vi "Table Stage Processor.vi"() -> ()   [LabVIEW 2018]
uses:
  Controls/QueueNames.ctl
  Controls/Queue Manager Actions.ctl
  Controls/MessagePacket.ctl
  Hardware Mfg/Thorlabs Translation Stages/Controls/Motion Translation Module Control.ctl
  Controls/Set Get Controls.ctl
  Controls/FGV Actions.ctl
  Hardware Mfg/Main Scan Processor Status.vi
  Controls/Translation Stage Types.ctl
  Hardware Mfg/Thorlabs Translation Stages/Controls/Translation Stage Cluster.ctl
panel:
  in  "error out":errorcluster
  out "Processor Error Out":errorcluster
  out "Cluster":cluster{"X":T1, "Y":T1, "Z":T1}
  out "Message":string
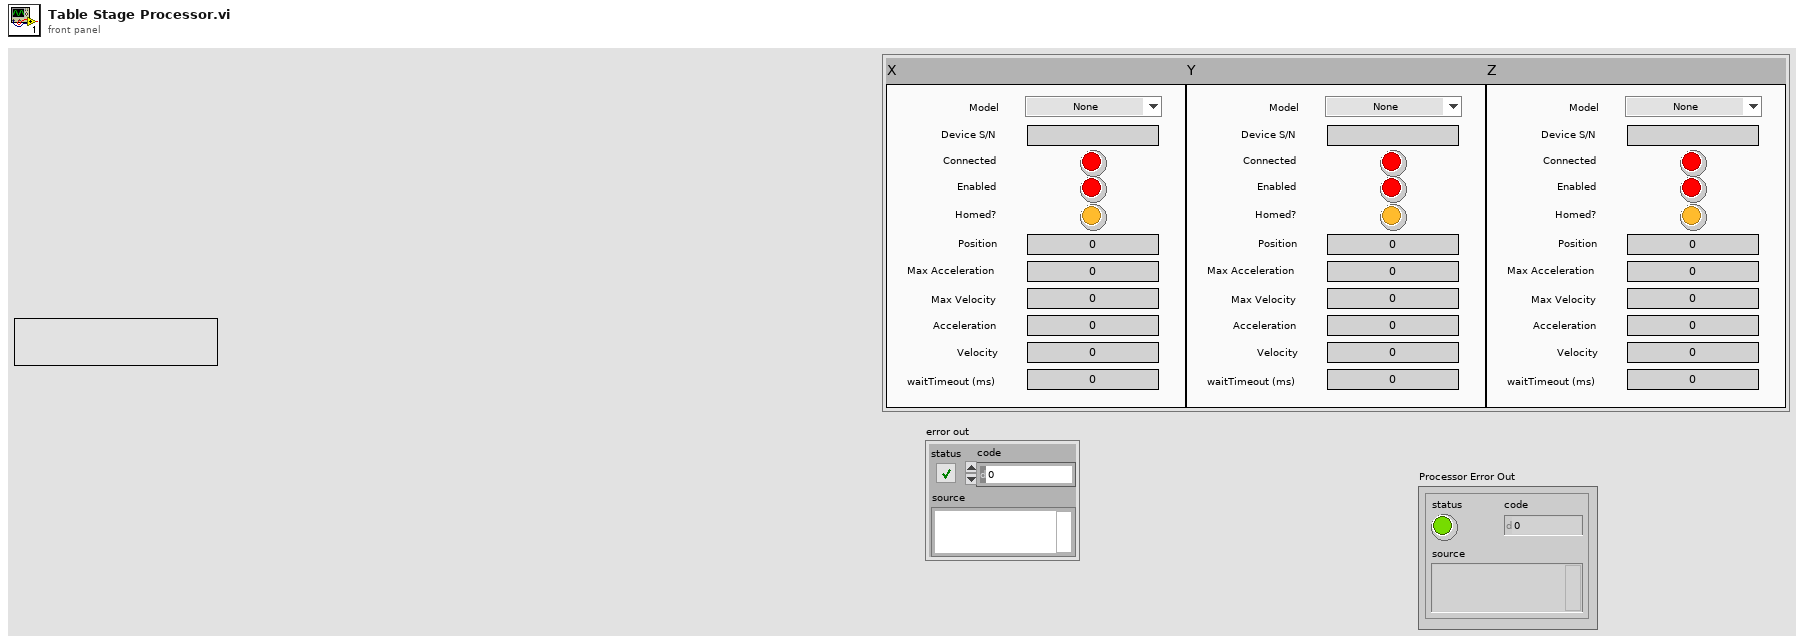
[diagram p1: front panel]
types:
  T1 = typedef "Translation Stage Cluster.ctl" = cluster{"Position":dbl, "Is.Enabled?":bool, "Is.Connected?":bool, "Device SN":string, "AccelerationMaximum":dbl, "VelocityMaximum":dbl, "Acceleration":dbl, "Velocity":dbl, "waitTimeout (ms)":i32, "Model":T2, "Is.Homed?":bool}
  T2 = typedef "Translation Stage Types.ctl" = enum16{"None", "Thorlabs LTS", "Thorlabs MLJ"}
  T3 = typedef "Queue Manager Actions.ctl" = enum16{"Init", "Enqueue", "Enqueue All", "Preview Queue", "Dequeue", "Get Status", "Flush Queue", "Flush All Queues", "Release All Queues", "Release Queue", "Enqueue at Opposite End"}
  T4 = typedef "MessagePacket.ctl" = cluster{"Message":string, "Parameter":variant}
  T5 = typedef "FGV Actions.ctl" = enum16{"Init", "Set", "Get", "Clear"}
  T6 = typedef "Set Get Controls.ctl" = enum16{"Set", "Get"}
  T7 = typedef "Motion Translation Module Control.ctl" = enum16{"Init", "Home", "Status", "Velocity/Accel", "Position", "Jog", "Stop", "Uninit", "Enable", "Disable"}
  T8 = typedef "QueueNames.ctl" = enum16{"Main GUI", "Main Scan Processor", "Main Display", "Main Table Stage GUI", "Main Table Stage Proc.", "Scan Engine", "Vibratome GUI", "Vibratome Processor", "Slice Engine", "Table Stage Processor"}
  T9 = cluster{"X Stage":T1, "Y Stage":T1, "Z Stage":T1}
  T10 = typedef "System Parameters.ctl" = cluster{"Optical /HW Parameters":cluster{"Focal Length [mm]":dbl, "Scan Lens EFL[mm]":dbl, "Tube Lens EFL[mm]":dbl, "Galvo V Range (+/-)":dbl, "Galvo Max Half Angle [Deg]":dbl, "Max Galvo Range[%]":dbl}, "Vibratome":cluster{"Z Bottom [mm]":dbl, "Pre Cut Dwell [s]":dbl, "Blade Frequency [RPM]":u16, "Slice Speed [mm/s]":dbl, "Post Cut Dwell [s]":dbl, "Ramp Time [s]":dbl, "Start X [mm]":dbl, "Start Y [mm]":dbl, "Slice Length [mm]":dbl, "Slice Axis":enum16{"X Axis", "Y Axis", "Z Axis"}, "Controller VISA Ref":refnum<visa-resource-name>}, "Table Stages":cluster{"X Stage":T1, "Y Stage":T1, "Z Stage":T1}, "Imaging Parameter":cluster{"Raster Scan Direction":T11, "Pixel Dwell Time [Clock Cycles]":u16, "Flyback Time [Clock Cycles]":u16, "XY Center [um]":cluster{"X":dbl, "Y":dbl}, "Pixel Step Size [um]":dbl, "XY Image Resolution":enum16{"32 x 32", "64 x 64", "128 x 128", "256 x 256", "512 x 512", "1024 x 1024", "2048 x 2048"}, "Custom":bool, "Custom Size":cluster{"X":u16, "Y":u16}, "Line Averages":u8}}
  T11 = typedef "Scan Direction.ctl" = enum16{"Uni Directional", "Bi Directional", "None"}
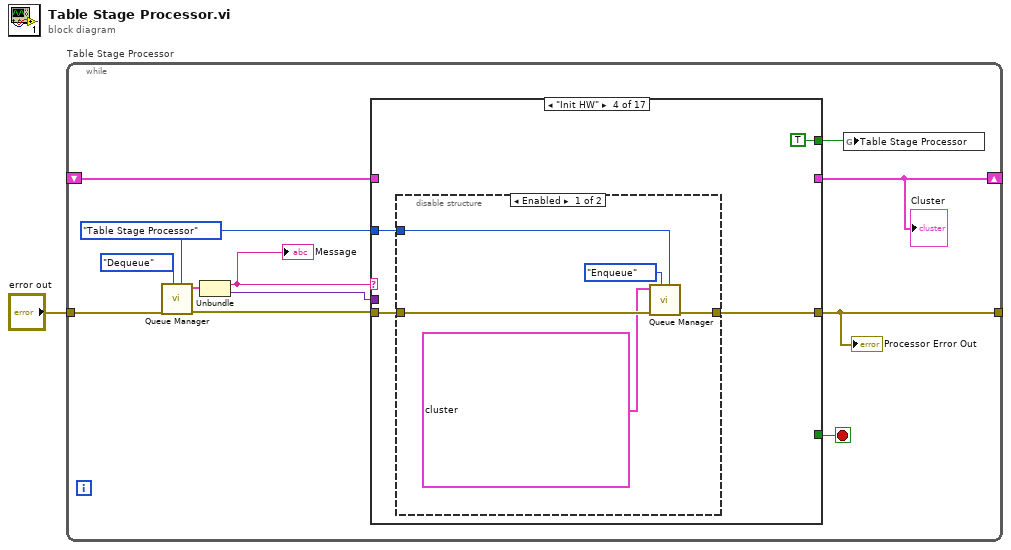
[diagram p0: block diagram]
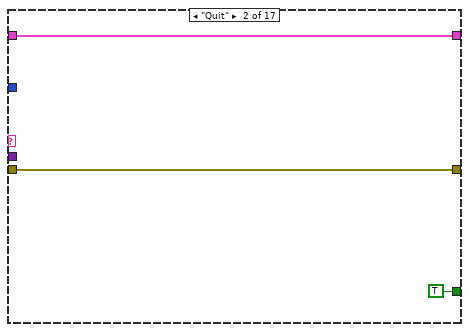
[diagram p3: hidden frame]
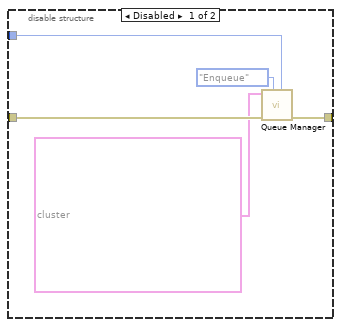
[diagram p5: hidden frame]
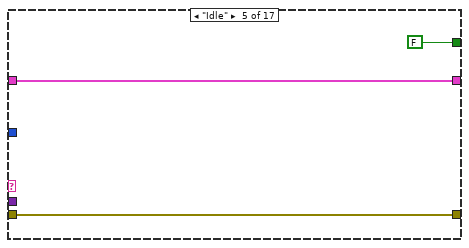
[diagram p7: hidden frame]
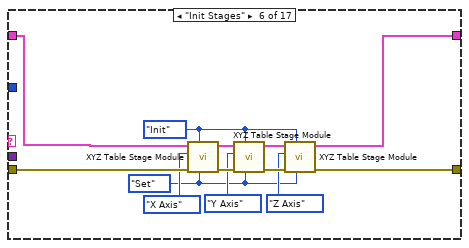
[diagram p8: hidden frame]
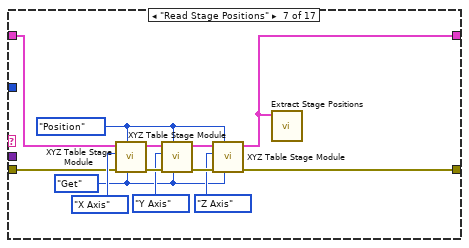
[diagram p9: hidden frame]
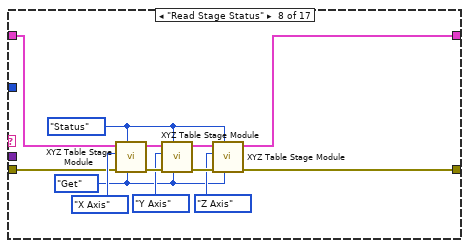
[diagram p10: hidden frame]
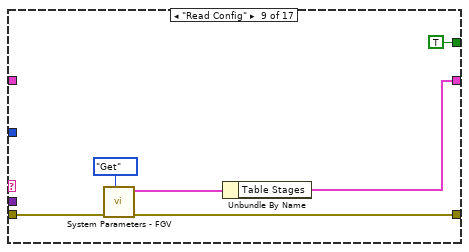
[diagram p11: hidden frame]
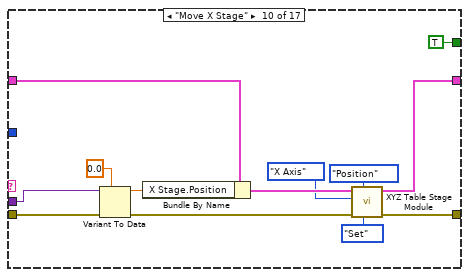
[diagram p12: hidden frame]
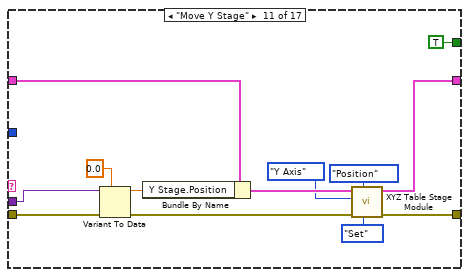
[diagram p13: hidden frame]
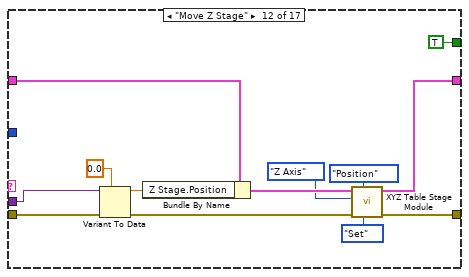
[diagram p14: hidden frame]
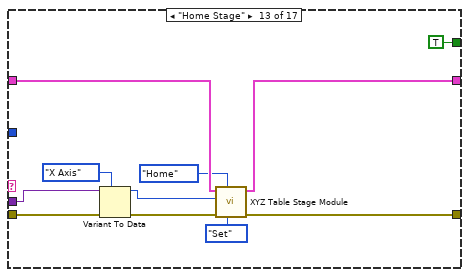
[diagram p15: hidden frame]
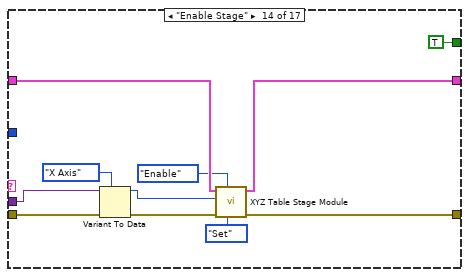
[diagram p16: hidden frame]
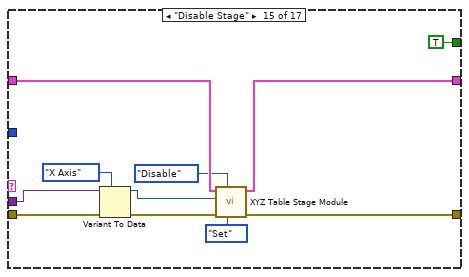
[diagram p17: hidden frame]
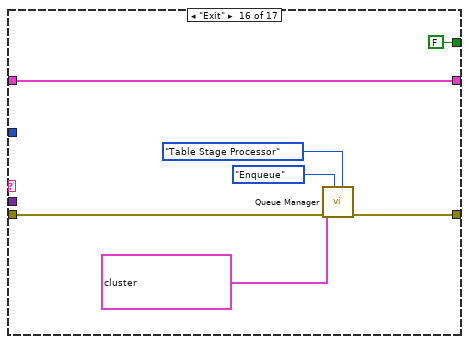
[diagram p18: hidden frame]
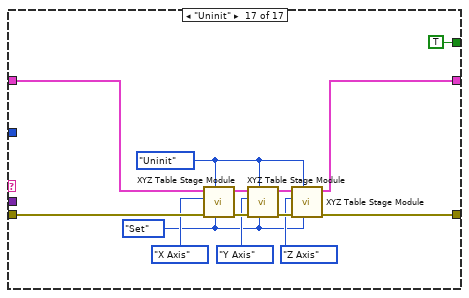
[diagram p19: hidden frame]
diagram:
  n1 = while "Table Stage Processor" {
    tunnel: "error out" -> [w12]
    tunnel: [w13] -> _
    shift-right: [w5] -> _
    shift-left: _ -> [w6]
    stop <- w8 stop-if-true
    w3 = QueueNames."Table Stage Processor" ("Queue Name")
    n2 = call "Queue Manager.vi"("Queue Name"=w3, "Action"=Queue_Manager_Actions."Dequeue", "Error In"=w12) -> ("Error Out"=w4:errorcluster, "Message Packet [Out]"=w11:T4)  [unwired: 4 in, 3 out]
    n3 = Unbundle(w11) -> ("Message"=w10:string, "Parameter"=w9:variant)
    "Message" <- w10
    n4 = case shown="\"Init HW\"" w10 {
      tunnel: w4 -> [w15 w17 w21 w31 w40 w52 w56 w69 w85 w98 w111 w124 w135 w146 w157 w163 w178]
      tunnel: [w15 w17 w20 w30 w40 w53 w64 w77 w83 w97 w110 w123 w134 w145 w156 w162 w166] -> w13
      tunnel: w9 -> [_ _ _ _ _ _ _ _ _ w95 w108 w121 w132 w143 w154 _ _]
      tunnel: [_ TRUE _ _ _ _ _ _ _ _ _ _ _ _ _ _ _] -> w8
      tunnel: [w14 w18 _ _ w39 w50 w54 w67 w84 w94 w107 w120 w128 w139 w150 w164 w172] -> w5
      tunnel: w6 -> [w14 w18 _ _ w39 w51 w55 w68 _ w90 w103 w116 w129 w140 w151 w164 w175]
      tunnel: w3 -> [_ _ w19 w29 _ _ _ _ _ _ _ _ _ _ _ _ _]
      tunnel: [_ _ _ TRUE FALSE _ _ _ TRUE TRUE TRUE TRUE TRUE TRUE TRUE FALSE TRUE] -> w2
      frame "Unknown", Default {
      }
      frame "Quit" {
      }
      frame "Init" {
        n5 = disable-structure shown="Enabled" {
          disable-tunnel: w21 -> [w26 w27]
          disable-tunnel: [w25 w27] -> w20
          disable-tunnel: w19 -> [w22 _]
          frame Disabled {
            n6 = call "Queue Manager.vi"("Queue Name"=w22, "Action"=Queue_Manager_Actions."Enqueue", "Error In"=w26, "Message Packet Array"=T4[] [{"Message"="Read Config", "Parameter"=variant}, {"Message"="Init Stage HW", "Parameter"=variant}, {"Message"="Read Stage Status", "Parameter"=variant}, {"Message"="Read Stage Positions", "Parameter"=variant}]) -> ("Error Out"=w25:errorcluster)  [unwired: 3 in, 4 out]
          }
          frame Enabled {
          }
        }
      }
      frame "Init HW" {
        n7 = disable-structure shown="Enabled" {
          disable-tunnel: w31 -> [w36 w37]
          disable-tunnel: [w35 w37] -> w30
          disable-tunnel: w29 -> [w32 _]
          frame Enabled {
            n8 = call "Queue Manager.vi"("Queue Name"=w32, "Action"=Queue_Manager_Actions."Enqueue", "Error In"=w36, "Message Packet Array"=T4[] [{"Message"="Read Config", "Parameter"=variant}, {"Message"="Init Stages", "Parameter"=variant}, {"Message"="Read Stage Status", "Parameter"=variant}, {"Message"="Read Stage Positions", "Parameter"=variant}, {"Message"="Idle", "Parameter"=variant}]) -> ("Error Out"=w35:errorcluster)  [unwired: 3 in, 4 out]
          }
          frame Disabled {
          }
        }
      }
      frame "Idle" {
      }
      frame "Init Stages" {
        w41 = Set_Get_Controls."Set" ("Set/Get")
        w47 = Motion_Translation_Module_Control."Init" ("Action")
        n9 = call "XYZ Table Stage Module.vi"("Set/Get"=w41, "Action"=w47, "Error In"=w52, "Axis"=enum16{"X Axis", "Y Axis", "Z Axis"}."X Axis", "Table Stages"=w51) -> ("Error Out"=w49:errorcluster, "Table Stages Out"=w46:T9)  [unwired: 5 in]
        n10 = call "XYZ Table Stage Module.vi"("Set/Get"=w41, "Action"=w47, "Error In"=w49, "Axis"=enum16{"X Axis", "Y Axis", "Z Axis"}."Y Axis", "Table Stages"=w46) -> ("Error Out"=w48:errorcluster, "Table Stages Out"=w45:T9)  [unwired: 5 in]
        n11 = call "XYZ Table Stage Module.vi"("Set/Get"=w41, "Action"=w47, "Error In"=w48, "Axis"=enum16{"X Axis", "Y Axis", "Z Axis"}."Z Axis", "Table Stages"=w45) -> ("Error Out"=w53:errorcluster, "Table Stages Out"=w50:T9)  [unwired: 5 in]
      }
      frame "Read Stage Positions" {
        w57 = Set_Get_Controls."Get" ("Set/Get")
        w63 = Motion_Translation_Module_Control."Position" ("Action")
        n12 = call "XYZ Table Stage Module.vi"("Set/Get"=w57, "Action"=w63, "Error In"=w56, "Axis"=enum16{"X Axis", "Y Axis", "Z Axis"}."X Axis", "Table Stages"=w55) -> ("Error Out"=w66:errorcluster, "Table Stages Out"=w62:T9)  [unwired: 5 in]
        n13 = call "XYZ Table Stage Module.vi"("Set/Get"=w57, "Action"=w63, "Error In"=w66, "Axis"=enum16{"X Axis", "Y Axis", "Z Axis"}."Y Axis", "Table Stages"=w62) -> ("Error Out"=w65:errorcluster, "Table Stages Out"=w61:T9)  [unwired: 5 in]
        n14 = call "XYZ Table Stage Module.vi"("Set/Get"=w57, "Action"=w63, "Error In"=w65, "Axis"=enum16{"X Axis", "Y Axis", "Z Axis"}."Z Axis", "Table Stages"=w61) -> ("Error Out"=w64:errorcluster, "Table Stages Out"=w54:T9)  [unwired: 5 in]
        n15 = call "Extract Stage Positions.vi"("Table Stages"=w54) -> ()  [unwired: 8 in, 3 out]
      }
      frame "Read Stage Status" {
        w70 = Set_Get_Controls."Get" ("Set/Get")
        w76 = Motion_Translation_Module_Control."Status" ("Action")
        n16 = call "XYZ Table Stage Module.vi"("Set/Get"=w70, "Action"=w76, "Error In"=w69, "Axis"=enum16{"X Axis", "Y Axis", "Z Axis"}."X Axis", "Table Stages"=w68) -> ("Error Out"=w79:errorcluster, "Table Stages Out"=w75:T9)  [unwired: 5 in]
        n17 = call "XYZ Table Stage Module.vi"("Set/Get"=w70, "Action"=w76, "Error In"=w79, "Axis"=enum16{"X Axis", "Y Axis", "Z Axis"}."Y Axis", "Table Stages"=w75) -> ("Error Out"=w78:errorcluster, "Table Stages Out"=w74:T9)  [unwired: 5 in]
        n18 = call "XYZ Table Stage Module.vi"("Set/Get"=w70, "Action"=w76, "Error In"=w78, "Axis"=enum16{"X Axis", "Y Axis", "Z Axis"}."Z Axis", "Table Stages"=w74) -> ("Error Out"=w77:errorcluster, "Table Stages Out"=w67:T9)  [unwired: 5 in]
      }
      frame "Read Config" {
        n19 = call "System Parameters - FGV.vi"("Actions"=FGV_Actions."Get", "Error In"=w85) -> ("Error Out"=w83:errorcluster, "System Parameters"=w82:T10)  [unwired: 8 in]
        n20 = Unbundle By Name(w82) -> ("Table Stages"=w84:T9)
      }
      frame "Move X Stage" {
        n21 = Variant To Data(error in=w98, type=0.0 ("Value"), Variant=w95) -> (data=w89:dbl, error out=w96:errorcluster)
        n22 = Bundle By Name(cluster=w90, "X Stage.Position"=w89) -> (w88:T9)
        n23 = call "XYZ Table Stage Module.vi"("Set/Get"=Set_Get_Controls."Set", "Action"=Motion_Translation_Module_Control."Position", "Error In"=w96, "Axis"=enum16{"X Axis", "Y Axis", "Z Axis"}."X Axis", "Table Stages"=w88) -> ("Error Out"=w97:errorcluster, "Table Stages Out"=w94:T9)  [unwired: 5 in]
      }
      frame "Move Y Stage" {
        n24 = Variant To Data(error in=w111, type=0.0 ("Value"), Variant=w108) -> (data=w102:dbl, error out=w109:errorcluster)
        n25 = Bundle By Name(cluster=w103, "Y Stage.Position"=w102) -> (w101:T9)
        n26 = call "XYZ Table Stage Module.vi"("Set/Get"=Set_Get_Controls."Set", "Action"=Motion_Translation_Module_Control."Position", "Error In"=w109, "Axis"=enum16{"X Axis", "Y Axis", "Z Axis"}."Y Axis", "Table Stages"=w101) -> ("Error Out"=w110:errorcluster, "Table Stages Out"=w107:T9)  [unwired: 5 in]
      }
      frame "Move Z Stage" {
        n27 = Variant To Data(error in=w124, type=0.0 ("Value"), Variant=w121) -> (data=w115:dbl, error out=w122:errorcluster)
        n28 = Bundle By Name(cluster=w116, "Z Stage.Position"=w115) -> (w114:T9)
        n29 = call "XYZ Table Stage Module.vi"("Set/Get"=Set_Get_Controls."Set", "Action"=Motion_Translation_Module_Control."Position", "Error In"=w122, "Axis"=enum16{"X Axis", "Y Axis", "Z Axis"}."Z Axis", "Table Stages"=w114) -> ("Error Out"=w123:errorcluster, "Table Stages Out"=w120:T9)  [unwired: 5 in]
      }
      frame "Home Stage" {
        n30 = Variant To Data(error in=w135, type=enum16{"X Axis", "Y Axis", "Z Axis"}."X Axis" ("Axis"), Variant=w132) -> (data=w130:enum16{"X Axis", "Y Axis", "Z Axis"}, error out=w133:errorcluster)
        n31 = call "XYZ Table Stage Module.vi"("Set/Get"=Set_Get_Controls."Set", "Action"=Motion_Translation_Module_Control."Home", "Error In"=w133, "Axis"=w130, "Table Stages"=w129) -> ("Error Out"=w134:errorcluster, "Table Stages Out"=w128:T9)  [unwired: 5 in]
      }
      frame "Enable Stage" {
        n32 = Variant To Data(error in=w146, type=enum16{"X Axis", "Y Axis", "Z Axis"}."X Axis" ("Axis"), Variant=w143) -> (data=w141:enum16{"X Axis", "Y Axis", "Z Axis"}, error out=w144:errorcluster)
        n33 = call "XYZ Table Stage Module.vi"("Set/Get"=Set_Get_Controls."Set", "Action"=Motion_Translation_Module_Control."Enable", "Error In"=w144, "Axis"=w141, "Table Stages"=w140) -> ("Error Out"=w145:errorcluster, "Table Stages Out"=w139:T9)  [unwired: 5 in]
      }
      frame "Disable Stage" {
        n34 = Variant To Data(error in=w157, type=enum16{"X Axis", "Y Axis", "Z Axis"}."X Axis" ("Axis"), Variant=w154) -> (data=w152:enum16{"X Axis", "Y Axis", "Z Axis"}, error out=w155:errorcluster)
        n35 = call "XYZ Table Stage Module.vi"("Set/Get"=Set_Get_Controls."Set", "Action"=Motion_Translation_Module_Control."Disable", "Error In"=w155, "Axis"=w152, "Table Stages"=w151) -> ("Error Out"=w156:errorcluster, "Table Stages Out"=w150:T9)  [unwired: 5 in]
      }
      frame "Exit" {
        n36 = call "Queue Manager.vi"("Queue Name"=QueueNames."Table Stage Processor", "Action"=Queue_Manager_Actions."Enqueue", "Error In"=w163, "Message Packet Array"=T4[] [{"Message"="Uninit", "Parameter"=variant}, {"Message"="Quit", "Parameter"=variant}]) -> ("Error Out"=w162:errorcluster)  [unwired: 3 in, 4 out]
      }
      frame "Uninit" {
        w167 = Set_Get_Controls."Set" ("Set/Get")
        w171 = Motion_Translation_Module_Control."Uninit" ("Action")
        n37 = call "XYZ Table Stage Module.vi"("Set/Get"=w167, "Action"=w171, "Error In"=w178, "Axis"=enum16{"X Axis", "Y Axis", "Z Axis"}."X Axis", "Table Stages"=w175) -> ("Error Out"=w176:errorcluster, "Table Stages Out"=w174:T9)  [unwired: 5 in]
        n38 = call "XYZ Table Stage Module.vi"("Set/Get"=w167, "Action"=w171, "Error In"=w176, "Axis"=enum16{"X Axis", "Y Axis", "Z Axis"}."Y Axis", "Table Stages"=w174) -> ("Error Out"=w177:errorcluster, "Table Stages Out"=w173:T9)  [unwired: 5 in]
        n39 = call "XYZ Table Stage Module.vi"("Set/Get"=w167, "Action"=w171, "Error In"=w177, "Axis"=enum16{"X Axis", "Y Axis", "Z Axis"}."Z Axis", "Table Stages"=w173) -> ("Error Out"=w166:errorcluster, "Table Stages Out"=w172:T9)  [unwired: 5 in]
      }
    }
    "Processor Error Out" <- w13
    "Cluster" <- w5
    n40 = global write "Main Scan Processor Status.vi" "Table Stage Processor"(w2) -> ()
  }
